vi "SetTrigger.vi"(8 "error in (no error)":errorcluster, 11 "ZWO_ASI in":refnum<class "ZWO_ASI.lvclass">) -> (0 "error out":errorcluster, 3 "ZWO_ASI out":refnum<class "ZWO_ASI.lvclass">)   [LabVIEW 2023, in "ZWO_ASI.lvlib" / "ZWO_ASI.lvclass"]
uses:
  ZWO_ASI.lvclass
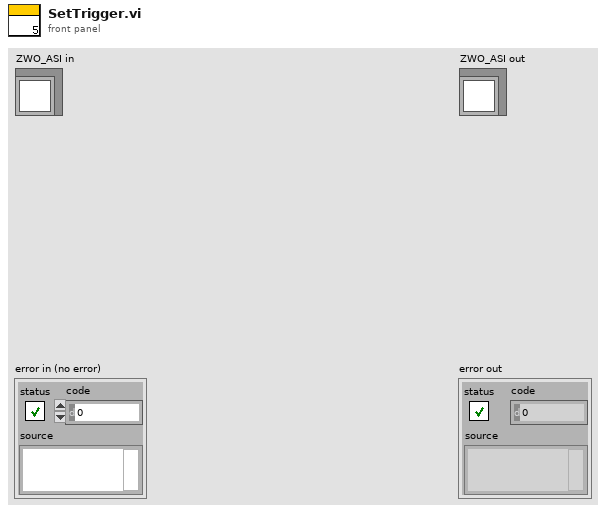
[diagram p1: front panel]
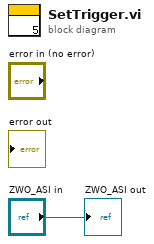
[diagram p0: block diagram]
diagram:
  "ZWO_ASI out" <- "ZWO_ASI in"
